vi "Create Special Complex Matrix.vi"(0 "matrix type":T1(ring), 1 "matrix size":i32, 3 "Input Vector1":cdb[](array[numeric]) format="%.2f", 4 "Input Vector2":cdb[](array[numeric]) format="%.2f") -> (5 "Special Matrix":T2, 6 "error":i32)   [LabVIEW 2010, in "NI_AALPro.lvlib"]
doc: "Generates a special matrix based on <B>matrix type</B>. The data types you wire to the <B>Input Vector2</B> and <B>Input Vector1</B> inputs determine the polymorphic instance to use."
uses:
  NI_AALPro.lvlib
  ComplexMatrix.ctl
  lvanlys.dll
  NI_Matrix.lvlib
panel:
  # "Create Special Complex Matrix"
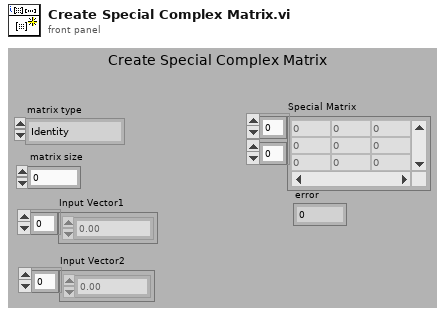
[diagram p1: front panel]
types:
  T1 = enum32{"Identity", "Diagonal", "Toepliz", "Vandermonde", "Companion"}
  T2 = typedef "NI_Matrix.lvlib/ComplexMatrix.ctl" = cdb[][]
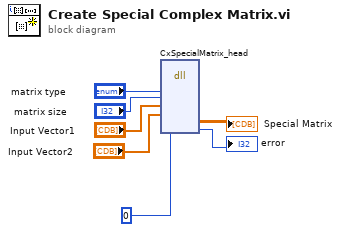
[diagram p0: block diagram]
diagram:
  n1 = dll-call lib="C:/Program Files/National Instruments/LabVIEW 2010/resource/lvanlys.*" fn="CxSpecialMatrix_head"("matrix type"="matrix type", "matrix size"="matrix size", "Input Vector1"="Input Vector1", "Input Vector2"="Input Vector2", 0) -> ("Special Matrix"=→"Special Matrix":T2, →"error":i32)  [unwired: 9 in, 2 out]
